vi "device_selector_panel.vi"(11 "error in (no error)":errorcluster) -> (4 "index":i32, 6 "chosen_sn":string, 8 "chosen_desc":string, 10 "cancel?":bool, 15 "error out":errorcluster)   [LabVIEW 2012]
doc: "Provides a simple, descriptive list (for user selection) of all USB based Performax devices attached to the PC. This is an EXAMPLE of an interface that might be used for collecting and displaying a list of devices to the user to choose frrom.\n\nProduced By:\n\nChristopher Lemieux\nKod Integrations, LLC\n4835 Marianne Drive\nMount Airy, MD 21771\nhttp://www.kodintegrations.com\nemail: clemieux@kodintegrations.com\nphone: (240) 687-1288"
uses:
  device_selector_panel_actions.vi
panel:
  in  "devices":i32(listbox)
  in  "cancel":bool
  in  "cont":bool
  # "Please choose a device from the list below"
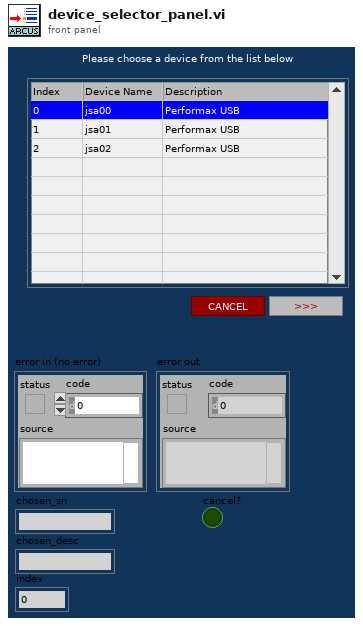
[diagram p1: front panel]
types:
  T1 = typedef "device_selector_panel_actions.vi" = enum16{"initialize", "processEvents", "validate", "continue", "cancel"}
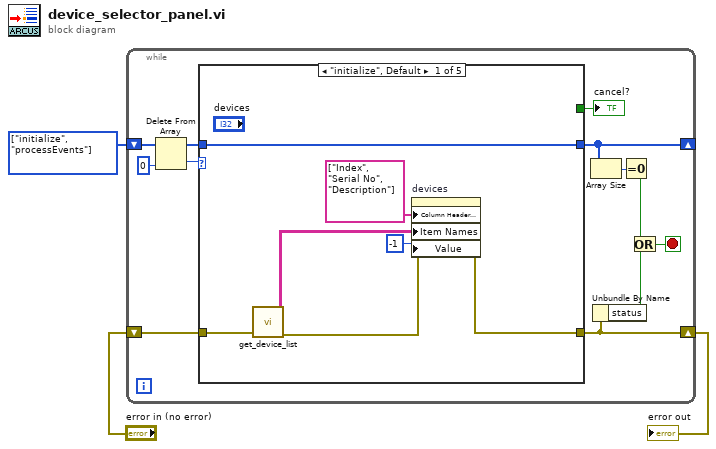
[diagram p0: block diagram]
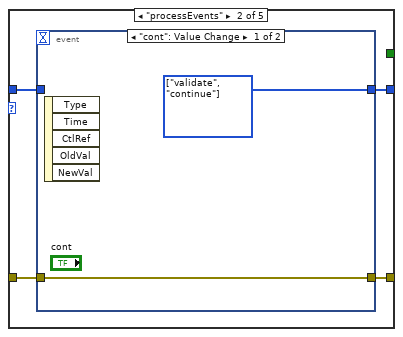
[diagram p2: hidden frame]
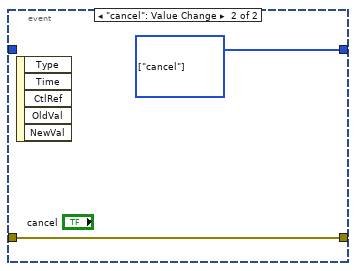
[diagram p3: hidden frame]
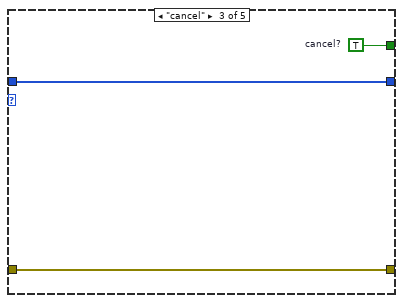
[diagram p4: hidden frame]
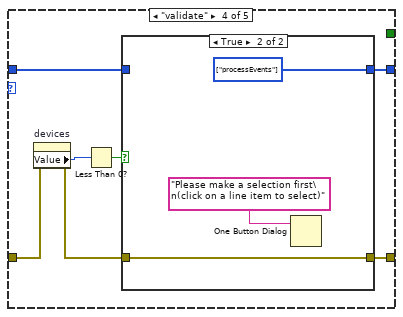
[diagram p5: hidden frame]
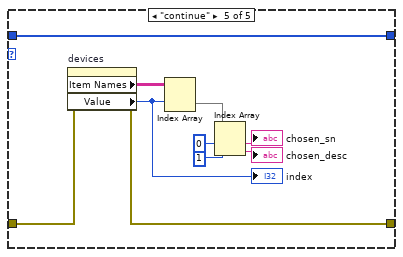
[diagram p7: hidden frame]
diagram:
  w3 = T1[] [enum."initialize", enum."processEvents"] items=["initialize", "processEvents", "validate", "continue", "cancel"]
  n1 = while {
    shift-right: [w10] -> _
    shift-left: w3 -> [w15]
    shift-right: [w8] -> w1
    shift-left: "error in (no error)" -> [w11]
    stop <- w5 stop-if-true
    n2 = Delete From Array(array=w15, index=0) -> (deleted portion=w13:T1, array with subset deleted=w12:T1[])  [unwired: 1 in]
    n3 = case shown="\"initialize\", Default" w13 {
      tunnel: [w17 w23 w32 w34 w55] -> w10
      tunnel: w12 -> [w17 w24 w32 w35 w55]
      tunnel: w11 -> [w19 w26 w31 w39 w47]
      tunnel: [w18 w25 w31 w37 w46] -> w8
      tunnel: [_ _ w33 _ _] -> w4
      frame "initialize", Default {
        n4 = call "get_device_list.vi"("error in (no error)"=w19) -> ("device_list"=w21:string[][], "error out"=w22:errorcluster)  [unwired: 13 in]
        n5 = property on="devices" class="MCListbox (strict)"(error in=w22, "Column Header Strings[]"=string[] ["Index", "Serial No", "Description"], "Item Names"=w21, "Value"=-1 ("devices")) -> (error out=w18:errorcluster)  [unwired: 1 in, 1 out]
      }
      frame "processEvents" {
        n6 = event shown="[0] \"cont\": Value Change" {
          selector: _ -> [_ _]
          dyn-events: _ -> [_ _]
          timeout: _ -> [_ _]
          tunnel: w26 -> [w28 w30]
          tunnel: [w28 w30] -> w25
          tunnel: w24 -> [_ _]
          tunnel: [w27 w29] -> w23
          event "cont": Value Change {
            w27 = T1[] [enum."validate", enum."continue"] items=["initialize", "processEvents", "validate", "continue", "cancel"]
            n7 = event-data() -> ()  [unwired: 1 in, 5 out]
          }
          event "cancel": Value Change {
            w29 = T1[] [enum."cancel"] items=["initialize", "processEvents", "validate", "continue", "cancel"]
            n8 = event-data() -> ()  [unwired: 1 in, 5 out]
          }
        }
      }
      frame "cancel" {
        w33 = TRUE  # cancel?
      }
      frame "validate" {
        n9 = property on="devices" class="MCListbox (strict)"(error in=w39) -> (error out=w38:errorcluster, "Value"=w40:i32)  [unwired: 1 in, 1 out]
        n10 = Less Than 0?(x=w40) -> (x < 0?=w36:bool)
        n11 = case shown="True" w36 {
          tunnel: [w42 w45] -> w37
          tunnel: w38 -> [w42 w45]
          tunnel: w35 -> [w41 _]
          tunnel: [w41 w43] -> w34
          frame False {
          }
          frame True {
            w43 = T1[] [enum."processEvents"] items=["initialize", "processEvents", "validate", "continue", "cancel"]
            n12 = One Button Dialog(message="Please make a selection first\n(click on a line item to select)") -> ()  [unwired: 1 in, 1 out]
          }
        }
      }
      frame "continue" {
        n13 = property on="devices" class="MCListbox (strict)"(error in=w47) -> (error out=w46:errorcluster, "Item Names"=w49:string[][], "Value"=w48:i32)  [unwired: 1 in, 1 out]
        "index" <- w48
        n14 = Index Array(array=w49, index (row)=w48) -> (element=w50:string[])  [unwired: 1 in]
        n15 = Index Array(array=w50, index #1=0 ("index"), index #2=1 ("index")) -> (element #1=→"chosen_sn":string, element #2=→"chosen_desc":string)
      }
    }
    "cancel?" <- w4
    n16 = Array Size(array=w10) -> (size(s)=w9:i32)
    n17 = Unbundle By Name(w8) -> ("status"=w6:bool)
    n18 = Equal To 0?(x=w9) -> (x = 0?=w7:bool)
    n19 = Or(x=w7, y=w6) -> (x .or. y?=w5:bool)
  }
  "error out" <- w1
